vi "simple_02.vi"() -> ()   [LabVIEW 2014]
uses:
  builds/LVTables/SQLite Packed/SQLite3LV.lvlibp/Cursor Class/property binding/column Text.vi
  builds/LVTables/SQLite Packed/SQLite3LV.lvlibp/SQLite3 Class/sqlite3.lvclass
  builds/LVTables/SQLite Packed/SQLite3LV.lvlibp/Cursor Class/cursor.lvclass
panel:
  out "sqlite_version()":string
  out "Array":string[](array[string])
  out "error out":errorcluster
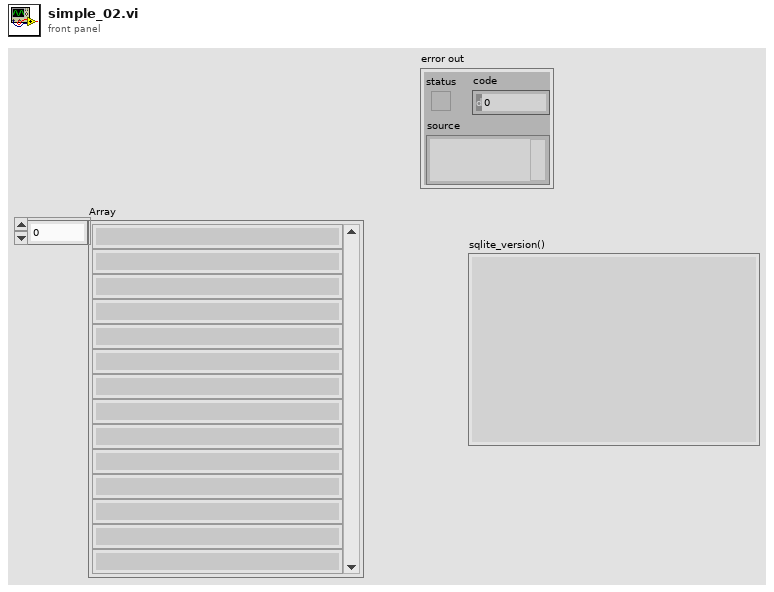
[diagram p1: front panel]
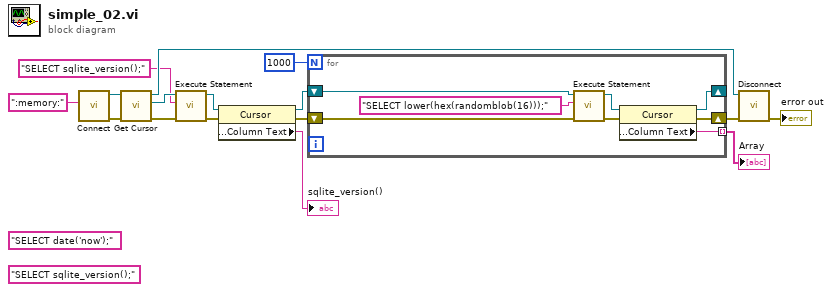
[diagram p0: block diagram]
diagram:
  (unwired) "SELECT sqlite_version();" ("SQL statement")
  (unwired) "SELECT date('now');" ("SQL statement")
  n1 = call "Connect.vi"("path"=":memory:") -> ("error out"=w13:errorcluster, "SQLite3LV Connection out"=w16:refnum<class "sqlite3.lvclass">)  [unwired: 9 in]
  n2 = call "Get Cursor.vi"("error in (no error)"=w13, "SQLite3LV Connection in"=w16) -> ("error out"=w8:errorcluster, "SQLite3LV Cursor"=w7:refnum<class "cursor.lvclass">, "SQLite3LV Connection out"=w15:refnum<class "sqlite3.lvclass">)  [unwired: 7 in]
  n3 = call "Execute Statement.vi"("error in (no error)"=w8, "SQL statement"="SELECT sqlite_version();", "SQLite3LV Cursor in"=w7) -> ("error out"=w4:errorcluster, "SQLite3LV Cursor out"=w5:refnum<class "cursor.lvclass">)  [unwired: 7 in]
  n4 = property class="Cursor"(reference=w5, error in=w4) -> (reference out=w3:refnum<class "cursor.lvclass">, error out=w2:errorcluster, "property binding:Column Text"=→"sqlite_version()":string)
  n5 = for {
    N: 1000 -> [_]
    shift-right: [w20] -> w14
    shift-left: w2 -> [w22]
    shift-right: [w18] -> _
    shift-left: w3 -> [w24]
    tunnel: [w17] -> w10 mode=indexing
    n6 = call "Execute Statement.vi"("error in (no error)"=w22, "SQL statement"="SELECT lower(hex(randomblob(16)));", "SQLite3LV Cursor in"=w24) -> ("error out"=w21:errorcluster, "SQLite3LV Cursor out"=w23:refnum<class "cursor.lvclass">)  [unwired: 7 in]
    n7 = property class="Cursor"(reference=w23, error in=w21) -> (reference out=w18:refnum<class "cursor.lvclass">, error out=w20:errorcluster, "property binding:Column Text"=w17:string)
  }
  "Array" <- w10
  n8 = call "Disconnect.vi"("error in (no error)"=w14, "SQLite3LV Connection in"=w15) -> ("error out"=→"error out":errorcluster)  [unwired: 9 in]
